vi "Launcher.vi"(7 "Open FP?":bool, 8 "error in (no error)":errorcluster, 9 "ICameraTestingUI":refnum<class "ICameraTestingUI.lvclass">, 10 "CameraInfo":T1, 11 "CameraTesting":refnum<class "CameraTesting.lvclass">) -> (0 "error out":errorcluster, 2 "Message Enqueuer out":refnum<class "Message Enqueuer.lvclass">)   [LabVIEW 2020, in "CameraTesting.lvlib" / "CameraTesting.lvclass"]
uses:
  CameraTesting.lvclass
  CameraTesting.lvclass/CameraTesting.ctl
  <vilib>/ActorFramework/Actor/Actor.lvclass
  CameraTesting Messages/Init Msg/Init Msg.lvclass
  <vilib>/ActorFramework/Message Enqueuer/Message Priority.ctl
  <vilib>/ActorFramework/Message Enqueuer/Message Enqueuer.lvclass
  C:/Program Files (x86)/National Instruments/LabVIEW 2020/vi.lib/ActorFramework/Actor/Actor.lvclass
  E:/GitHub/Evaluation_Test/Labview/src/CameraTestingApp/CameraTesting/CameraTesting/CameraTesting.lvclass
  E:/GitHub/Evaluation_Test/Labview/src/CameraTestingApp/ICameraTesting/ICameraTesting/ICameraTesting.lvclass
  Camera/ICamera/ICamera/ICamera.lvclass
  ICameraTestingUI/ICameraTestingUI/ICameraTestingUI.lvclass
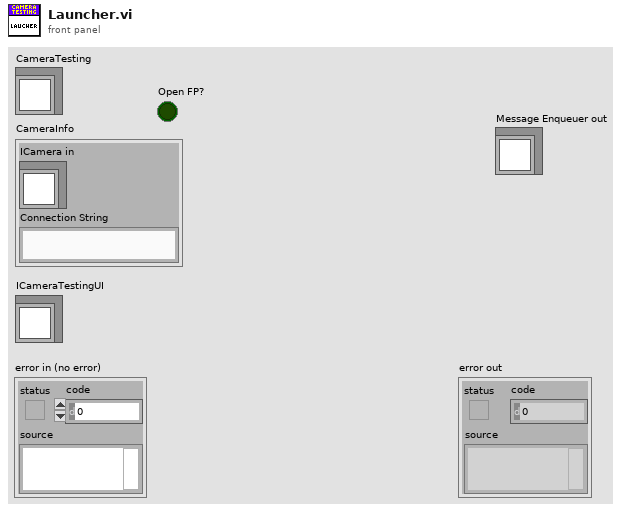
[diagram p1: front panel]
types:
  T1 = cluster{"ICamera in":refnum<class "ICamera.lvclass">, "Connection String":string}
  T2 = typedef "Actor Framework.lvlib/Message Enqueuer.lvclass/Message Priority.ctl" = enum16{"Low", "Normal", "High"}
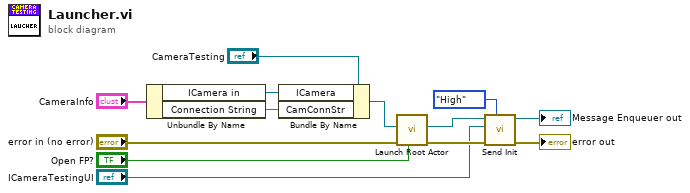
[diagram p0: block diagram]
diagram:
  n1 = Unbundle By Name("CameraInfo") -> ("ICamera in"=w3:refnum<class "ICamera.lvclass">, "Connection String"=w2:string)
  n2 = Bundle By Name(cluster="CameraTesting", "ICamera"=w3, "CamConnStr"=w2) -> (w1:refnum<class "CameraTesting.lvclass">)
  n3 = call <vilib>:"Launch Root Actor.vi"("Open Actor Core front panel? (F)"="Open FP?", "error in (no error)"="error in (no error)", "Actor"=w1) -> ("error out"=w12:errorcluster, "Actor's Enqueuer"=w13:refnum<class "Message Enqueuer.lvclass">)  [unwired: 7 in]
  n4 = call "Send Init.vi"("Message Priority (Normal)"=Message_Priority."High", "error in (no error)"=w12, "ICameraTestingUI.lvlib:ICameraTestingUI.lvclass"="ICameraTestingUI", "Message Enqueuer"=w13) -> ("error out"=→"error out":errorcluster, "Message Enqueuer out"=→"Message Enqueuer out":refnum<class "Message Enqueuer.lvclass">)  [unwired: 6 in]
